vi "Create.vi"(8 "error in (no error)":errorcluster, 10 "Account Database":refnum<class "Account Database.lvclass">) -> (0 "error out":errorcluster, 3 "ATM Controller out":refnum<class "ATM Controller.lvclass">)   [LabVIEW 2020, in "ATM Controller.lvclass"]
uses:
  ATM Controller.lvclass
  Account Database/Account Database.lvclass
  ATM Controller.lvclass/ATM Controller.ctl
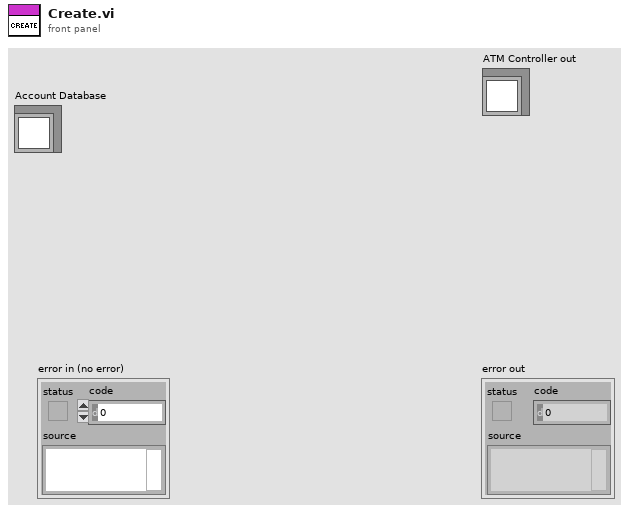
[diagram p1: front panel]
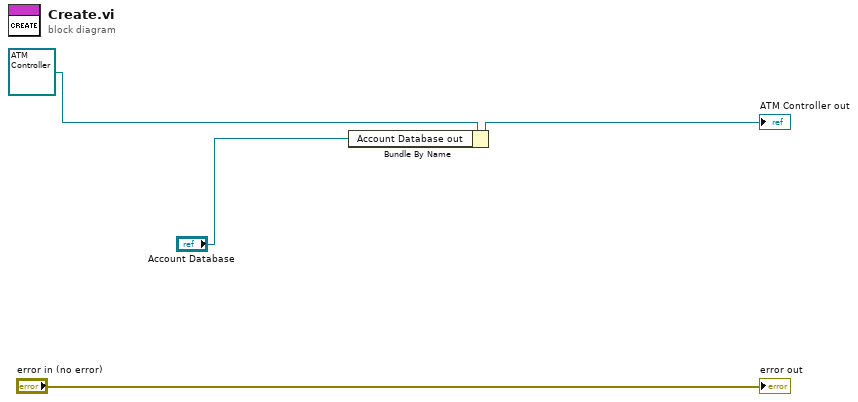
[diagram p0: block diagram]
diagram:
  n1 = Bundle By Name(cluster=refnum<class "ATM Controller.lvclass"> refnum ("ATM Controller in"), "Account Database out"="Account Database") -> (→"ATM Controller out":refnum<class "ATM Controller.lvclass">)
  "error out" <- "error in (no error)"
